vi "Write Exec Reentrancy Type.vi"(8 "error in (no error)":errorcluster, 9 "Execution:Inline SubVI":bool, 10 "Execution:Reentrancy Type":T1(ring), 11 "file path":path) -> (0 "error out":errorcluster)   [LabVIEW 2022 SP3]
uses:
  66691eb3-70af-41bc-86bd-00228d7174ee.vi
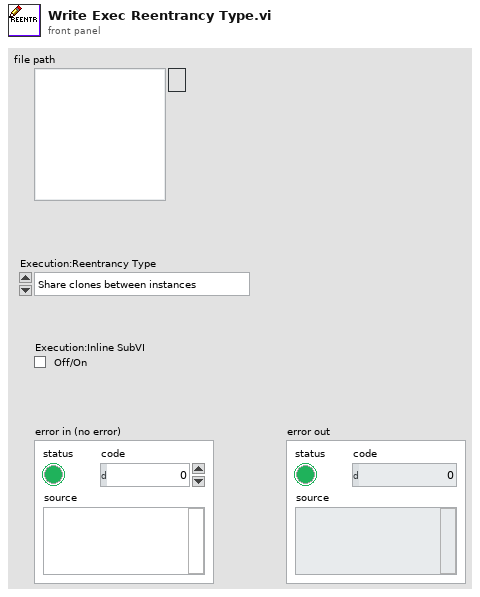
[diagram p1: front panel]
types:
  T1 = enum16{"Share clones between instances", "Preallocate clone for each instance"}
  T2 = enum32{"Invalid", "Standard", "Closed", "Hidden", "Minimized", "Maximized"}
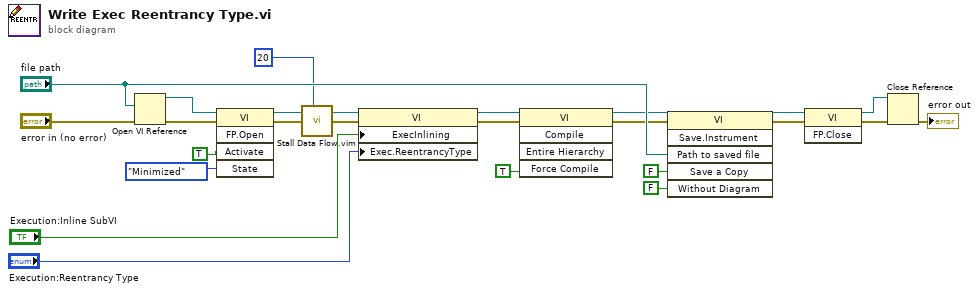
[diagram p0: block diagram]
diagram:
  n1 = Open VI Reference(vi path="file path", error in (no error)="error in (no error)") -> (vi reference=w24:refnum<vi>, error out=w18:errorcluster)  [unwired: 4 in]
  n2 = invoke class="VI" method="FP.Open"(reference=w24, error in=w18, "Activate"=TRUE ("Activate?"), "State"=T2."Minimized") -> (reference out=w19:refnum<vi>, error out=w17:errorcluster)  [unwired: 1 in, 3 out]
  n3 = call "Stall Data Flow.vim"("value in"=w17, "milliseconds to wait"=u32 20) -> ("value out"=w2:errorcluster)  [unwired: 1 out]
  n4 = property class="VI"(reference=w19, error in=w2, "ExecInlining"="Execution:Inline SubVI", "Exec.ReentrancyType"="Execution:Reentrancy Type") -> (reference out=w21:refnum<vi>, error out=w20:errorcluster)
  n5 = invoke class="VI" method="Compile"(reference=w21, error in=w20, "Force Compile"=TRUE ("Force Compile (T)")) -> (reference out=w10:refnum<vi>, error out=w9:errorcluster)  [unwired: 2 in, 3 out]
  n6 = invoke class="VI" method="Save.Instrument"(reference=w10, error in=w9, "Path to saved file"="file path", "Save a Copy"=FALSE, "Without Diagram"=FALSE) -> (reference out=w8:refnum<vi>, error out=w7:errorcluster)  [unwired: 1 in, 4 out]
  n7 = invoke class="VI" method="FP.Close"(reference=w8, error in=w7) -> (reference out=w16:refnum<vi>, error out=w15:errorcluster)  [unwired: 1 in, 1 out]
  n8 = Close Reference(reference=w16, error in (no error)=w15) -> (error out=→"error out":errorcluster)
